vi "Test_TerminalEnabledState_EqualToZero_Disabled.vi"(8 "error in (no error)":errorcluster, 11 "TestCase in":refnum<class "TestTransport.lvclass">) -> (0 "error out":errorcluster, 3 "TestCase out":refnum<class "TestTransport.lvclass">)   [LabVIEW 2017, in "TestTransport.lvclass"]
uses:
  TestTransport.lvclass
  TerminalEnabledStateBinding/TerminalEnabledStateBinding.lvclass
panel:
  out "An I32 Terminal":i32
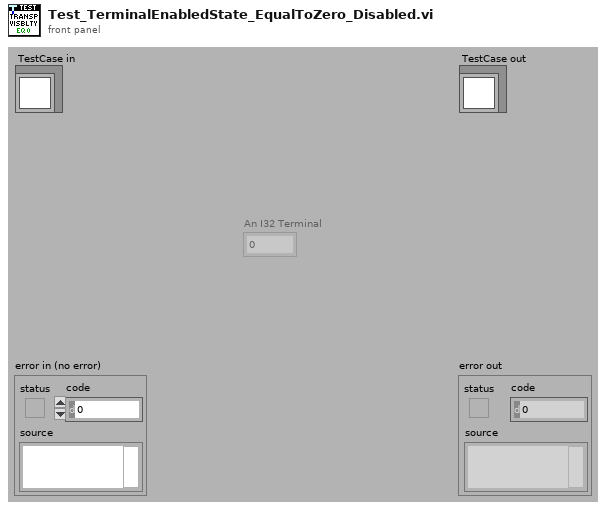
[diagram p1: front panel]
types:
  T1 = enum8{"Enabled", "Disabled", "Disabled and Grayed Out"}
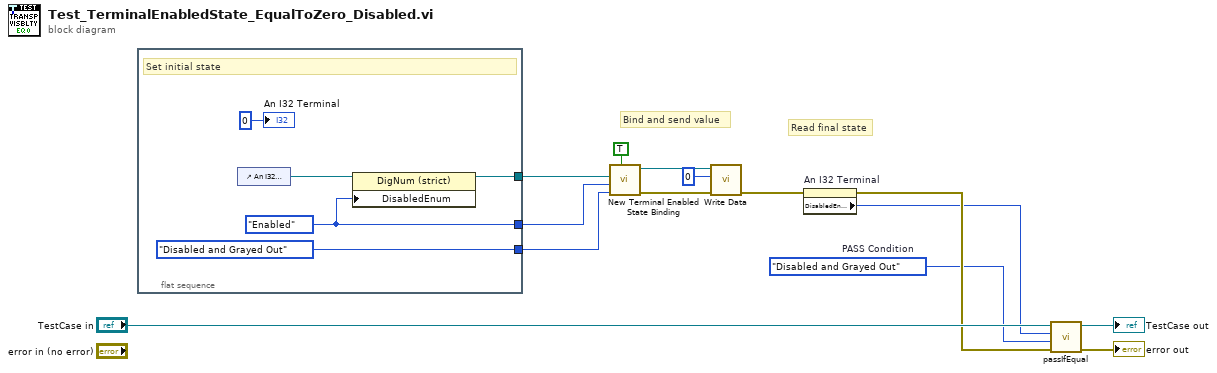
[diagram p0: block diagram]
diagram:
  w1 = T1."Disabled and Grayed Out"  # PASS Condition
  # "Bind and send value"
  # "Read final state"
  n1 = flat-sequence {
    tunnel: [w17] -> w8
    tunnel: [T1."Disabled and Grayed Out" ("Disabled")] -> w4
    tunnel: [w15] -> w3
    frame #0 {
      w15 = T1."Enabled" ("Disabled")
      # "Set initial state"
      n2 = control-ref of="An I32 Terminal"() -> (w18:refnum<vi>)
      n3 = property class="DigNum (strict)"(reference=w18, "DisabledEnum"=w15) -> (reference out=w17:refnum<vi>)  [unwired: 1 in, 1 out]
      "An I32 Terminal" <- 0 ("An I32 Terminal")
    }
  }
  n4 = call "New Terminal Enabled State Binding.vi"("Initial State (T)"=TRUE, "FALSE State (Disabled and Grayed Out)"=w4, "TRUE State (Enabled)"=w3, "Control"=w8) -> ("error out"=w7:errorcluster, "TerminalEnabledStateBinding Out"=w11:refnum<class "TerminalEnabledStateBinding.lvclass">)  [unwired: 6 in]
  n5 = call-dynamic "Write Data.vi"("error in (no error)"=w7, "Value"=0, "TerminalEnabledStateBinding In"=w11) -> ("error out"=w9:errorcluster)  [unwired: 7 in, 1 out]
  n6 = property on="An I32 Terminal" class="DigNum (strict)"(error in=w9) -> (error out=w6:errorcluster, "DisabledEnum"=w5:T1)  [unwired: 1 in, 1 out]
  n7 = call-dynamic "passIfEqual.vi"("error in (no error)"=w6, "y"=w1, "x"=w5, "TestCase in"="TestCase in") -> ("error out"=→"error out":errorcluster, "TestCase out"=→"TestCase out":refnum<class "TestTransport.lvclass">)  [unwired: 6 in]
